vi "todatacluster.vi"(10 "ROI":T3, 11 "Images":T5) -> (3 "data":T1)   [LabVIEW 2013]
uses:
  ROIStartfromCam_typdef.ctl
  classicROI_typDef.ctl
  analysis_data_typdef.ctl
  <vilib>/vision/Image Controls.llb/IMAQ Image.ctl
  dataTypdef.ctl
  MagAnalysis_Online.lvclass
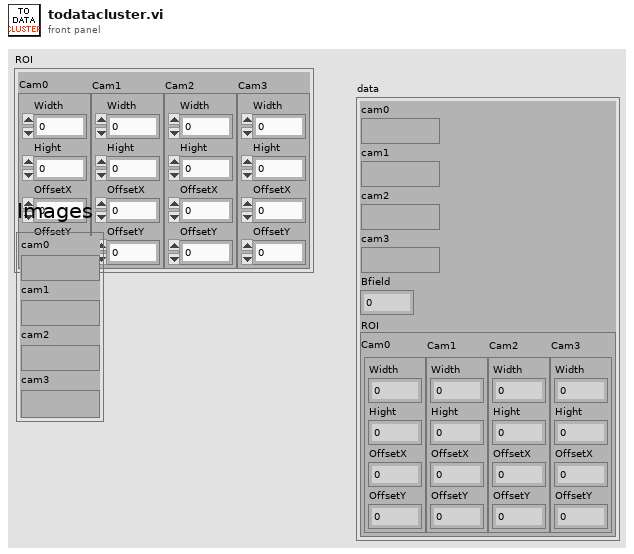
[diagram p1: front panel]
types:
  T1 = typedef "dataTypdef.ctl" = cluster{"cam0":T2, "cam1":T2, "cam2":T2, "cam3":T2, "Bfield":dbl, "ROI":T3}
  T2 = typedef "IMAQ Image.ctl" = refnum<image>
  T3 = typedef "ROIStartfromCam_typdef.ctl" = cluster{"Cam0":T4, "Cam1":T4, "Cam2":T4, "Cam3":T4}
  T4 = typedef "classicROI_typDef.ctl" = cluster{"Width":dbl, "Hight":dbl, "OffsetX":dbl, "OffsetY":dbl}
  T5 = typedef "MagAnalysis_Online.lvclass/analysis_data_typdef.ctl" = cluster{"cam0":T2, "cam1":T2, "cam2":T2, "cam3":T2}
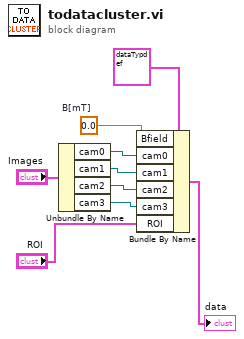
[diagram p0: block diagram]
diagram:
  w5 = 0.0  # B[mT]
  n1 = Unbundle By Name("Images") -> ("cam0"=w8:T2, "cam1"=w7:T2, "cam2"=w6:T2, "cam3"=w1:T2)
  n2 = Bundle By Name(cluster=T1 {"cam0"=refnum, "cam1"=refnum, "cam2"=refnum, "cam3"=refnum, "Bfield"=0.0, "ROI"={"Cam0"={"Width"=0.0, "Hight"=0.0, "OffsetX"=0.0, "OffsetY"=0.0}, "Cam1"={"Width"=0.0, "Hight"=0.0, "OffsetX"=0.0, "OffsetY"=0.0}, "Cam2"={"Width"=0.0, "Hight"=0.0, "OffsetX"=0.0, "OffsetY"=0.0}, "Cam3"={"Width"=0.0, "Hight"=0.0, "OffsetX"=0.0, "OffsetY"=0.0}}} ("data"), "Bfield"=w5, "cam0"=w8, "cam1"=w7, "cam2"=w6, "cam3"=w1, "ROI"="ROI") -> (→"data":T1)
